vi "readInXMLNative.vi"(8 "error in (no error)":errorcluster, 10 "scriptEventXML":refnum<k20>, 11 "ScriptEvent in":refnum<class "ScriptEvent.lvclass">) -> (0 "error out":errorcluster, 3 "ScriptEvent out":refnum<class "ScriptEvent.lvclass">)   [LabVIEW 2009, in "Tools.lvlib" / "Scripting.lvlib" / "ScriptEvent.lvclass"]
uses:
  ScriptEvent.lvclass
  <vilib>/xml/Close Reference(Node).vi
  <vilib>/xml/NI_XML.lvlib
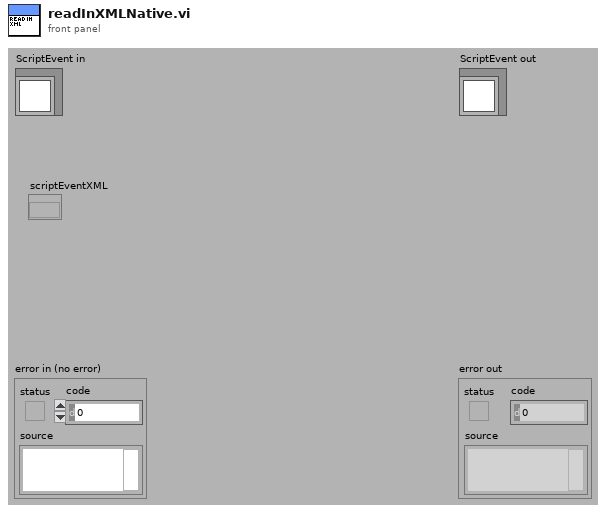
[diagram p1: front panel]
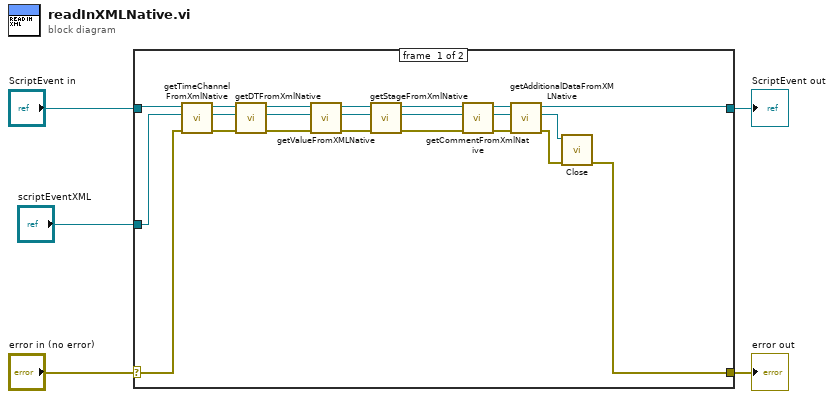
[diagram p0: block diagram]
diagram:
  n1 = case shown="No Error" "error in (no error)" {
    selector: "error in (no error)" -> [w7 w29]
    tunnel: [w6 w29] -> w4
    tunnel: [w19 w28] -> w2
    tunnel: "ScriptEvent in" -> [w27 w28]
    tunnel: "scriptEventXML" -> [w26 _]
    frame #0 {
      n2 = call "getTimeChannelFromXmlNative.vi"("error in (no error)"=w7, "eventXML"=w26, "ScriptEvent in"=w27) -> ("error out"=w24:errorcluster, "eventXML out"=w13:refnum<k20>, "ScriptEvent out"=w25:refnum<class "ScriptEvent.lvclass">)  [unwired: 6 in]
      n3 = call "getDTFromXmlNative.vi"("error in (no error)"=w24, "eventXML"=w13, "ScriptEvent in"=w25) -> ("error out"=w15:errorcluster, "eventXML out"=w14:refnum<k20>, "ScriptEvent out"=w23:refnum<class "ScriptEvent.lvclass">)  [unwired: 6 in]
      n4 = call-dynamic "getValueFromXMLNative.vi"("error in (no error)"=w15, "eventXML"=w14, "ScriptEvent in"=w23) -> ("error out"=w16:errorcluster, "eventXML out"=w10:refnum<k20>, "ScriptEvent out"=w22:refnum<class "ScriptEvent.lvclass">)  [unwired: 6 in]
      n5 = call "getStageFromXmlNative.vi"("error in (no error)"=w16, "eventXML"=w10, "ScriptEvent in"=w22) -> ("error out"=w17:errorcluster, "eventXML out"=w12:refnum<k20>, "ScriptEvent out"=w21:refnum<class "ScriptEvent.lvclass">)  [unwired: 6 in]
      n6 = call "getCommentFromXmlNative.vi"("error in (no error)"=w17, "eventXML"=w12, "ScriptEvent in"=w21) -> ("error out"=w18:errorcluster, "eventXML out"=w11:refnum<k20>, "ScriptEvent out"=w20:refnum<class "ScriptEvent.lvclass">)  [unwired: 6 in]
      n7 = call-dynamic "getAdditionalDataFromXMLNative.vi"("error in (no error)"=w18, "eventXML"=w11, "ScriptEvent in"=w20) -> ("error out"=w9:errorcluster, "eventXML out"=w8:refnum<k20>, "ScriptEvent out"=w19:refnum<class "ScriptEvent.lvclass">)  [unwired: 6 in]
      n8 = call-poly <vilib>:"Close.vi"("error in (no error)"=w9, "node"=w8) -> ("error out"=w6:errorcluster)  [unwired: 7 in]
    }
    frame #1 {
    }
  }
  "error out" <- w4
  "ScriptEvent out" <- w2
